vi "Read Min Max Data.vi"(8 "error in (no error)":errorcluster, 10 "Channel (1:1)":u16(ring)=1 items=["1"=1, "2"=2, "3"=3, "4"=4, "5"=5, "6"=6, "7"=7, "8"=8, "9"=9, "10"=10, "11"=11, "12"=12, "13"=13, "14"=14, "15"=15, "16"=16, "A (Control Input)"=17], 11 "VISA resource name":refnum<visa-resource-name>) -> (0 "error out":errorcluster, 1 "Min Value":dbl min=0.0 max=63200000.0 step=1e-05 format="%^.5e", 2 "Max Value":dbl min=0.0 max=63200000.0 step=1e-05 format="%^.5e", 3 "VISA resource name out":refnum<visa-resource-name>)   [LabVIEW 2018, in "Lake Shore 372.lvlib"]
doc: "Returns the channel's min/max readings."
uses:
  Lake Shore 372.lvlib
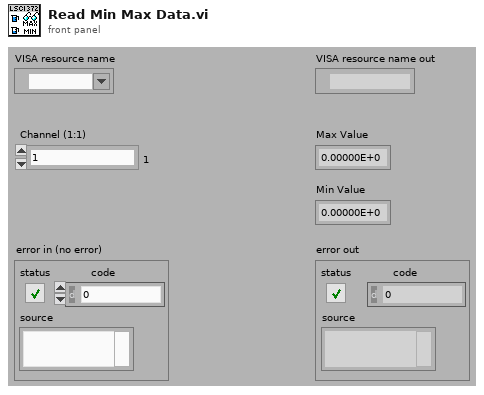
[diagram p1: front panel]
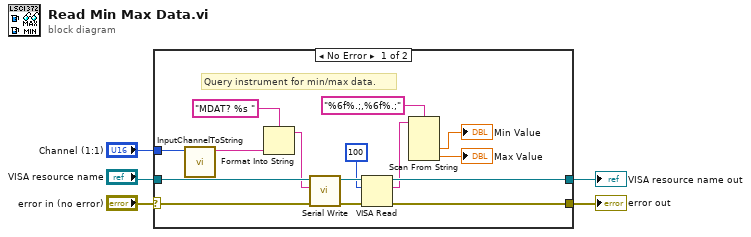
[diagram p0: block diagram]
diagram:
  n1 = case shown="No Error" "error in (no error)" {
    selector: "error in (no error)" -> [w7 w21]
    tunnel: "VISA resource name" -> [w17 w22]
    tunnel: [w16 w21] -> w4
    tunnel: [w15 w22] -> w3
    tunnel: "Channel (1:1)" -> [w9 _]
    frame No Error {
      # "Query instrument for min/max data."
      n2 = call "InputChannelToString.vi"("Channel (1)"=w9) -> ("Channel Str"=w8:string)  [unwired: 10 in]
      n3 = Format Into String(format string="MDAT? %s ", w8) -> (resulting string=w10:string)  [unwired: 2 in, 1 out]
      n4 = call "Serial Write.vi"("error in (no error)"=w7, "Write Buffer (\"\")"=w10, "VISA resource name"=w17) -> ("error out"=w19:errorcluster, "VISA resource name out"=w20:refnum<visa-resource-name>)  [unwired: 6 in, 1 out]
      n5 = VISA Read(VISA resource name=w20, byte count=100, error in (no error)=w19) -> (VISA resource name out=w15:refnum<visa-resource-name>, read buffer=w6:string, error out=w16:errorcluster)  [unwired: 1 out]
      n6 = Scan From String(format string="%6f%.;,%6f%.;", input string=w6) -> (output 1=→"Min Value":dbl, output 2=→"Max Value":dbl)  [unwired: 4 in, 3 out]
    }
    frame Error {
    }
  }
  "error out" <- w4
  "VISA resource name out" <- w3
